vi "TracePoint_NewCamera.vi"(8 "error in (no error)":errorcluster, 10 "new camera":T1, 11 "Qbus":refnum<class "Qbus.lvclass">) -> (0 "error out":errorcluster)   [LabVIEW 2017, in "IrAcquisition.lvlib"]
uses:
  <vilib>/addons/InsightCM/Devices/Shared/Ir/IrAcquisition/IrAcquisition.lvlib
  <vilib>/addons/Qbus/Qbus.lvclass
  <vilib>/addons/InsightCM/Devices/Shared/Ir/IrAcquisition/controls/camera.ctl
  <vilib>/userdefined/High Color/IMAQdx.ctl
  <vilib>/vision/Image Controls.llb/IMAQ Image.ctl
  <vilib>/addons/PointValueMap/controls/PointMap.ctl
  <vilib>/addons/TraceLogger/TraceLogger.lvlib
  <vilib>/addons/PointValueMap/PointValueMap.lvlib
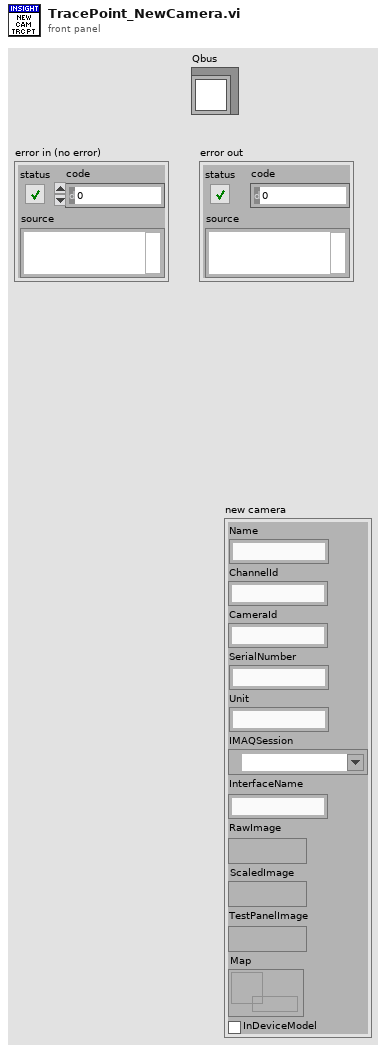
[diagram p1: front panel]
types:
  T1 = typedef "IrAcquisition.lvlib/camera.ctl" = cluster{"Name":string, "ChannelId":string, "CameraId":string, "SerialNumber":string, "Unit":string, "IMAQSession":T2, "InterfaceName":string, "RawImage":T3, "ScaledImage":T3, "TestPanelImage":T3, "Map":T4, "InDeviceModel":bool}
  T2 = typedef "IMAQdx.ctl" = refnum<k21>
  T3 = typedef "IMAQ Image.ctl" = refnum<image>
  T4 = typedef "PointValueMap.lvlib/PointMap.ctl" = refnum<data-value>
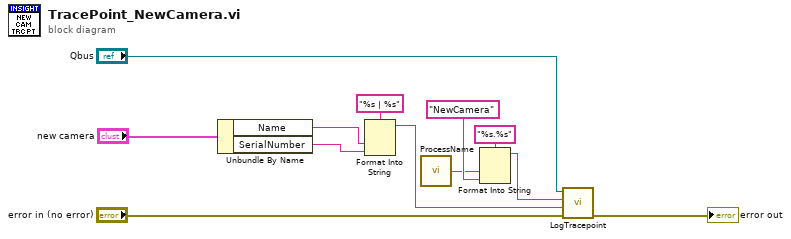
[diagram p0: block diagram]
diagram:
  n1 = Unbundle By Name("new camera") -> ("Name"=w2:string, "SerialNumber"=w3:string)
  n2 = Format Into String(format string="%s | %s", w2, w3) -> (resulting string=w5:string)  [unwired: 2 in, 1 out]
  n3 = call <vilib>:"ProcessName.vi"() -> ("process name"=w4:string)  [unwired: 5 in]
  n4 = Format Into String(format string="%s.%s", w4, "NewCamera" ("tracepoint")) -> (resulting string=w7:string)  [unwired: 2 in, 1 out]
  n5 = call <vilib>:"LogTracepoint.vi"("error in (no error)"="error in (no error)", "log string"=w5, "tracepoint"=w7, "qbus in"="Qbus") -> ("error out"=→"error out":errorcluster)  [unwired: 6 in, 1 out]
